vi "Camera_GUI.vi"(10 "stop 2":refnum<vi>, 11 "GUI_cluster":T1={"Sub Panel"=refnum, "GUIdevice"="Bella_LP_Mode", "CtlRef"=refnum, "user event out"=refnum}) -> ()   [LabVIEW 2011]
uses:
  GUI_Template/GUI_master/tcp_new_data_event.ctl
  GUI_Template/GUI_master/tcp new data cluster.ctl
  Controls/GUI_cluster.ctl
  Controls/eventtypdef.ctl
  <vilib>/vision/Image Controls.llb/IMAQ Image.ctl
panel:
  out "tcp data event":T2
  in  "trigger::2":bool caption="Trigger"
  in  "gain::2":dbl=0.001 caption="gain" min=0.0 max=10.0 format="%_1p"
  out "image::2":T3(plugin-control) caption="Mode1"
  in  "exposure::2":dbl=0.001 caption="exposure" min=0.001 max=1.0 format="%_1p"
  out "GUIdevice 2":string="Bella_LP_Mode"
  in  "stop":bool
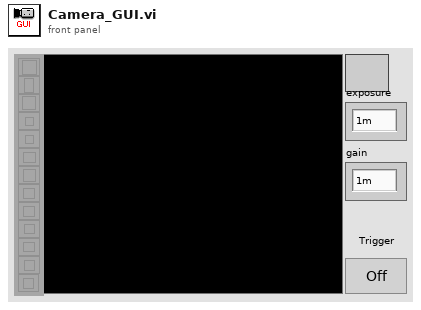
[diagram p1: front panel]
types:
  T1 = typedef "GUI_cluster.ctl" = cluster{"Sub Panel":refnum<vi>, "GUIdevice":string, "CtlRef":refnum<vi>, "user event out":refnum<user-event>}
  T2 = typedef "tcp_new_data_event.ctl" = refnum<user-event>
  T3 = typedef "IMAQ Image.ctl" = refnum<image>
  T4 = typedef "eventtypdef.ctl" = cluster{"label":string, "Sub Panel":refnum<vi>, "CtlRef":refnum<vi>, "This VI":refnum<vi>}
  T5 = typedef "tcp new data cluster.ctl" = cluster{"EventEnum":enum16{"new data", "connection status update"}, "Device name":string}
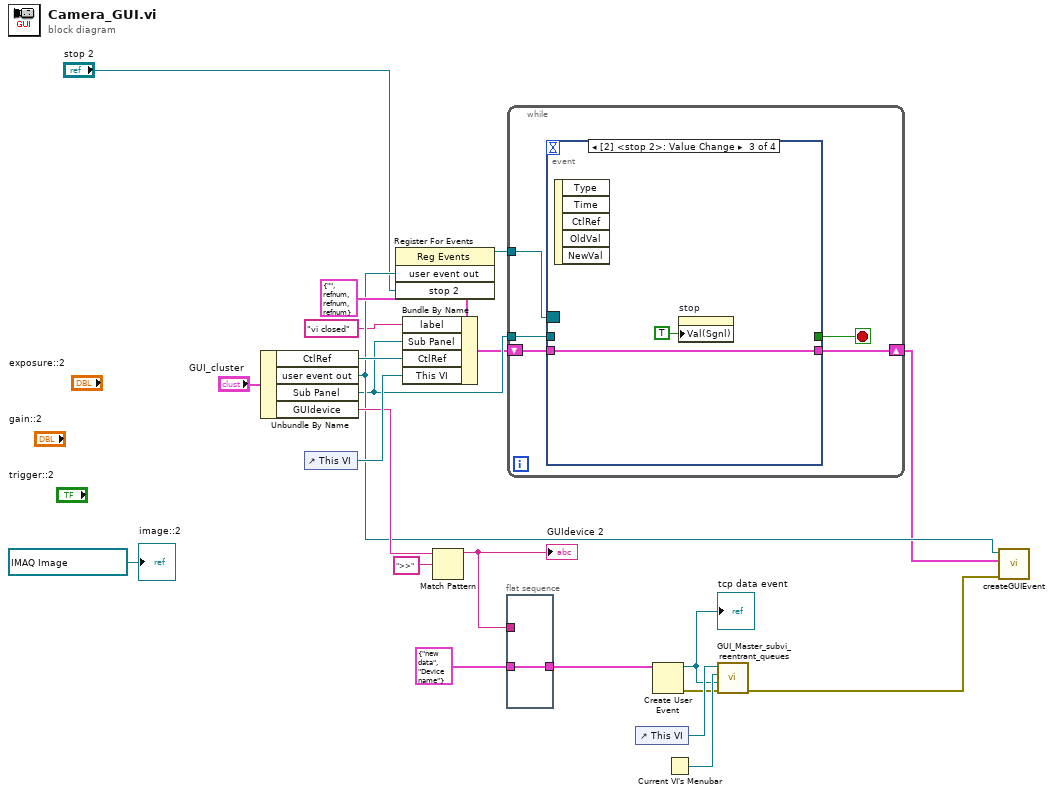
[diagram p0: block diagram]
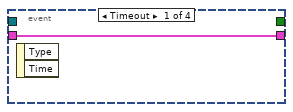
[diagram p2: hidden frame]
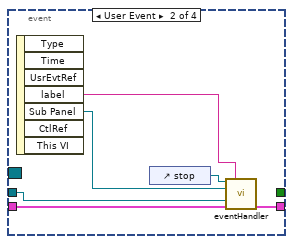
[diagram p3: hidden frame]
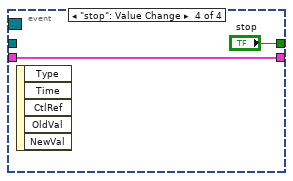
[diagram p4: hidden frame]
diagram:
  n1 = Unbundle By Name("GUI_cluster") -> ("CtlRef"=w15:refnum<vi>, "user event out"=w9:refnum<user-event>, "Sub Panel"=w8:refnum<vi>, "GUIdevice"=w12:string)
  n2 = control-ref of="This VI"() -> (w14:refnum<vi>)
  n3 = register-events(w9, "stop 2") -> (reference out=w10:refnum<event-registration>)  [unwired: 2 in, 1 out]
  n4 = Bundle By Name(cluster=T4 {"label"="", "Sub Panel"=refnum, "CtlRef"=refnum, "This VI"=refnum} ("event data"), "label"="vi closed", "Sub Panel"=w8, "CtlRef"=w15, "This VI"=w14) -> (w6:T4)
  n5 = Match Pattern(string=w12, regular expression=">>") -> (before substring=w2:string)  [unwired: 1 in, 3 out]
  "GUIdevice 2" <- w2
  n6 = flat-sequence {
    tunnel: T5 {"EventEnum"=enum."new data", "Device name"="Device name"} ("New Event") -> [w23]
    tunnel: [w23] -> w3
    tunnel: w2 -> [_]
    frame #0 {
    }
  }
  n7 = while {
    tunnel: w10 -> [w28]
    tunnel: w8 -> [w26]
    shift-right: [w24] -> w5
    shift-left: w6 -> [w25]
    stop <- w27 stop-if-true
    n8 = event shown="[2] <stop 2>: Value Change" {
      selector: w28 -> [_ _ _ _]
      dyn-events: _ -> [_ _ _ _]
      timeout: _ -> [_ _ _ _]
      tunnel: [_ _ _ "stop"] -> w27
      tunnel: w26 -> [_ w32 _ _]
      tunnel: w25 -> [w29 w31 w36 w38]
      tunnel: [w29 w30 w36 w38] -> w24
      event Timeout {
        n9 = event-data() -> ()  [unwired: 1 in, 2 out]
      }
      event User Event {
        n10 = event-data() -> ("label"=w35:string, "Sub Panel"=w34:refnum<vi>)  [unwired: 1 in, 5 out]
        n11 = control-ref of="stop"() -> (w33:refnum<vi>)
        n12 = call "eventHandler.vi"("Boolean in"=w33, "label"=w35, "Sub Panel 2"=w34, "Sub Panel"=w32, "event data in"=w31) -> ("event data out"=w30:T4)  [unwired: 10 in]
      }
      event Value Change {
        n13 = event-data() -> ()  [unwired: 1 in, 5 out]
        n14 = property on="stop" class="Bool (strict)"("Val(Sgnl)"=TRUE ("Value (Signaling)")) -> ()  [unwired: 2 in, 2 out]
      }
      event "stop": Value Change {
        n15 = event-data() -> ()  [unwired: 1 in, 5 out]
      }
    }
  }
  n16 = control-ref of="This VI"() -> (w22:refnum<vi>)
  n17 = Create User Event(user event datatype=w3) -> (user event=w18:refnum<user-event>, error out=w19:errorcluster)  [unwired: 1 in]
  "tcp data event" <- w18
  n18 = Current VI's Menubar() -> (w21:refnum<k9>)
  n19 = call "GUI_Master_subvi_reentrant_queues.vi"("error in (no error)"=w19, "tcp data event"=w18, "Caller menu reference"=w21, "Caller VI ref"=w22) -> ("error out"=w13:errorcluster)  [unwired: 7 in]
  n20 = call "createGUIEvent.vi"("error in (no error)"=w13, "event data"=w5, "User Event in"=w9) -> ()  [unwired: 9 in]
  "image::2" <- T3 refnum ("New Image")
